vi "Test_Draw_Polylines_ARGB.vi"(8 "error in (no error)":errorcluster, 11 "Test Case In":refnum<class "Image.lvclass">) -> (0 "error out":errorcluster, 3 "Test Case Out":refnum<class "Image.lvclass">)   [LabVIEW 2020, in "g_ar_toolkit.test.lvlib" / "Image.lvclass"]
uses:
  Image.lvclass
  Image.lvclass/Image.ctl
  g_ar_toolkit.image/g_ar_toolkit.image.lvlib
  g_ar_toolkit.image/CreateEmptyImageARGB.vi
  g_ar_toolkit.image/ARGB Colour.ctl
  g_ar_toolkit.image/Image Size (Fixed).ctl
  g_ar_toolkit.image/Image Point (Fixed).ctl
  g_ar_toolkit.image/Line Type.ctl
  g_ar_toolkit.image/Poly Lines Shape Draw Mode.ctl
  4993e8ee-a06a-463a-9684-69129f64d5ce.vi
panel:
  out "Picture":picture
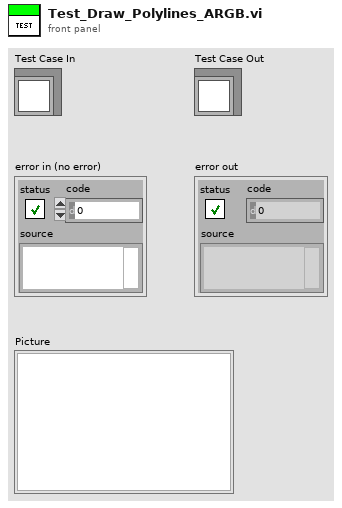
[diagram p1: front panel]
types:
  T1 = typedef "g_ar_toolkit.image.lvlib/Poly Lines Shape Draw Mode.ctl" = enum16{"Close Points", "Leave Points Open"}
  T2 = typedef "g_ar_toolkit.image.lvlib/Image Point (Fixed).ctl" = cluster{"x":i32, "y":i32}
  T3 = typedef "g_ar_toolkit.image.lvlib/Line Type.ctl" = enum8{"FILLED", "LINE_4", "LINE_8", "LINE_AA"}
  T4 = typedef "g_ar_toolkit.image.lvlib/ARGB Colour.ctl" = cluster{"Alpha":u8, "RGB":u32}
  T5 = typedef "g_ar_toolkit.image.lvlib/Image Size (Fixed).ctl" = cluster{"Width":u16, "Height":u16}
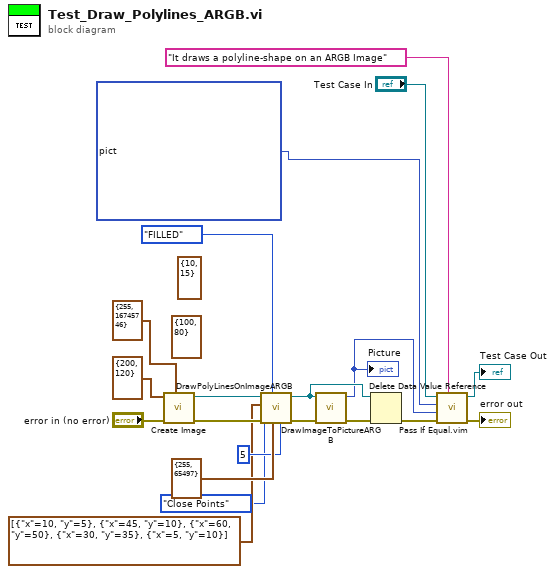
[diagram p0: block diagram]
diagram:
  (unwired) T2 {"x"=100, "y"=80} ("Point B")
  (unwired) T2 {"x"=10, "y"=15} ("Centre")
  n1 = call-poly "Create Image.vi"("Colour (Default: Black)"=T4 {"Alpha"=255, "RGB"=16745746}, "error in (no error)"="error in (no error)", "Preallocated Image Size (Default: 0,0)"=T5 {"Width"=200, "Height"=120}) -> ("error out"=w13:errorcluster, "New ARGB Image"=w14:refnum<data-value>)  [unwired: 7 in]
  n2 = call "DrawPolyLinesOnImageARGB.vi"("Thickness (Default: 1)"=u16 5, "ARGB Colour"=T4 {"Alpha"=255, "RGB"=65497}, "OpenCV Line Type (Default LINE_8)"=Line_Type."FILLED", "error in (no error)"=w13, "Draw Mode (Default: Close Points)"=Poly_Lines_Shape_Draw_Mode."Close Points", "Points"=T2[] [{"x"=10, "y"=5}, {"x"=45, "y"=10}, {"x"=60, "y"=50}, {"x"=30, "y"=35}, {"x"=5, "y"=10}], "ARGB Image"=w14) -> ("error out"=w11:errorcluster, "ARGB Image (Duplicate)"=w12:refnum<data-value>)  [unwired: 3 in]
  n3 = call "DrawImageToPictureARGB.vi"("error in (no error)"=w11, "ARGB Image Source"=w12) -> ("error out"=w10:errorcluster, "Picture"=w5:picture)  [unwired: 8 in]
  "Picture" <- w5
  n4 = Delete Data Value Reference(data value reference=w12, error in=w10) -> (error out=w16:errorcluster)  [unwired: 1 out]
  n5 = call "Pass If Equal.vim"("Description"="It draws a polyline-shape on an ARGB Image", "error in (no error)"=w16, "Actual"=w5, "Expected"=picture bytes[72030] ("Picture"), "LUnit Test Case In"="Test Case In") -> ("error out"=→"error out":errorcluster, "LUnit Test Case Out"=→"Test Case Out":refnum<class "Image.lvclass">)  [unwired: 5 in]
